vi "Enable New Station.vi"(8 "error in (no error)":errorcluster, 11 "OPC Server in":refnum<class "OPC Server.lvclass">) -> (0 "error out":errorcluster, 3 "OPC Server out":refnum<class "OPC Server.lvclass">)   [LabVIEW 2021, in "OPC Server.lvlib" / "OPC Server.lvclass"]
uses:
  OPC Server.lvclass
  OPC Server.lvclass/OPC Server.ctl
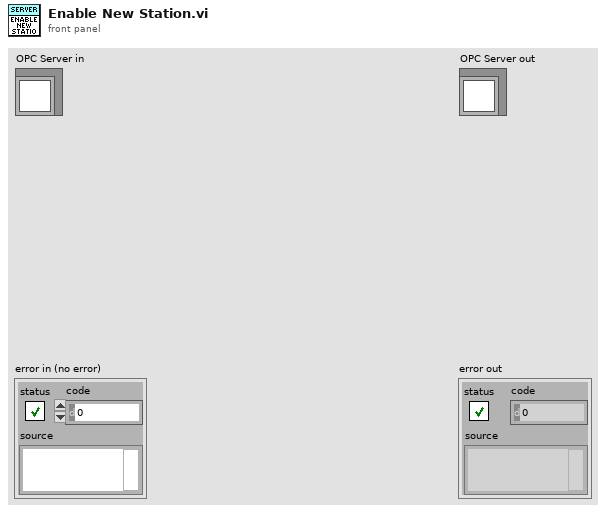
[diagram p1: front panel]
types:
  T1 = enum8{"Enabled", "Disabled", "Disabled and Grayed Out"}
  T2 = typedef "LVComboBoxStrsAndValuesArrayTypeDef.ctl" = cluster{"String":string, "Value":string}[]
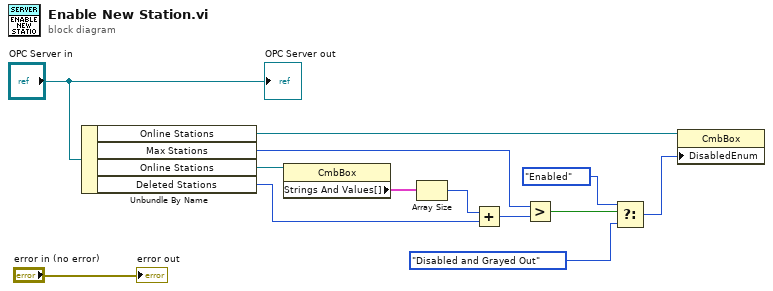
[diagram p0: block diagram]
diagram:
  n1 = Unbundle By Name("OPC Server in") -> ("Online Stations"=w5:refnum<vi>, "Max Stations"=w10:i32, "Online Stations"=w12:refnum<vi>, "Deleted Stations"=w8:u32)
  n2 = property class="CmbBox"(reference=w12) -> ("Strings And Values[]"=w11:T2)  [unwired: 1 in, 2 out]
  n3 = Array Size(array=w11) -> (size(s)=w9:i32)
  n4 = Add(x=w9, y=w8) -> (x+y=w7:u32)
  n5 = Greater?(x=w10, y=w7) -> (0:w4:bool)
  n6 = Select(t=T1."Enabled" ("Disabled"), s=w4, f=T1."Disabled and Grayed Out" ("Disabled")) -> (s? t:f=w1:T1)
  n7 = property class="CmbBox"(reference=w5, "DisabledEnum"=w1) -> ()  [unwired: 1 in, 2 out]
  "error out" <- "error in (no error)"
  "OPC Server out" <- "OPC Server in"
